vi "Create Unique File.vi"(8 "error in (no error)":errorcluster, 11 "appended path":path) -> (0 "error out":errorcluster, 3 "Byte Stream File out":refnum<file>)   [LabVIEW 2020, in "Global_logger.lvlib"]
uses:
  Global_logger.lvlib
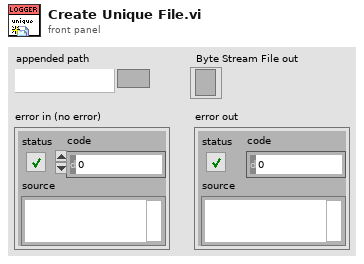
[diagram p1: front panel]
types:
  T1 = enum16{"open", "replace", "create", "open or create", "replace or create", "replace or create with confirmation"}
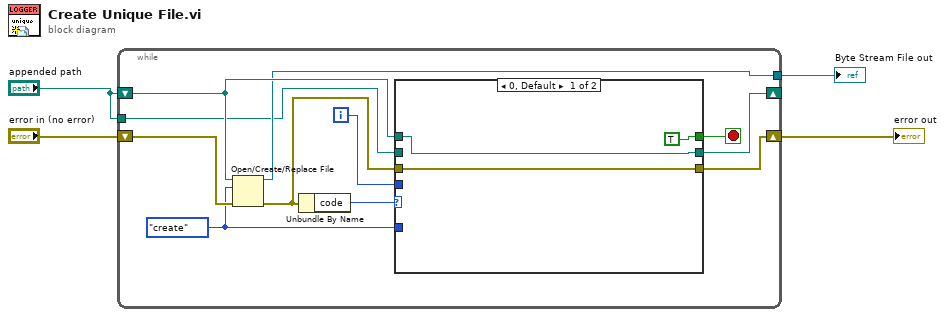
[diagram p0: block diagram]
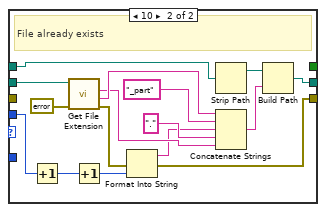
[diagram p2: hidden frame]
diagram:
  n1 = while {
    tunnel: [w7] -> w4
    shift-right: [w13] -> w3
    shift-left: "error in (no error)" -> [w15]
    shift-right: [w8] -> _
    shift-left: "appended path" -> [w11]
    tunnel: "appended path" -> [w5]
    i -> [w6]
    stop <- w9 stop-if-true
    w10 = T1."create" ("operation (0:open)")
    n2 = Open/Create/Replace File(file path (use dialog)=w11, error in=w15, operation (0:open)=w10) -> (refnum out=w7:refnum<file>, error out=w12:errorcluster)  [unwired: 3 in, 1 out]
    n3 = Unbundle By Name(w12) -> ("code"=w14:i32)
    n4 = case shown="0, Default" w14 {
      tunnel: [w18 w22] -> w13
      tunnel: w12 -> [w18 _]
      tunnel: w11 -> [w16 w27]
      tunnel: w10 -> [_ _]
      tunnel: [TRUE _] -> w9
      tunnel: [w16 w28] -> w8
      tunnel: w6 -> [_ w25]
      tunnel: w5 -> [_ w20]
      frame 0, Default {
      }
      frame 10 {
        # "File already exists"
        n5 = Increment(x=w25) -> (x+1=w21:i32)
        n6 = call <vilib>:"Get File Extension.vi"("error in (no error)"=errorcluster {"status"=FALSE, "code"=0, "source"=""} ("error in"), "file"=w20) -> ("error out"=w23:errorcluster, "filename without extension"=w33:string, "lowercase file extension"=w30:string)  [unwired: 5 in, 2 out]
        n7 = Increment(x=w21) -> (x+1=w19:i32)
        n8 = Format Into String(error in=w23, w19) -> (resulting string=w24:string, error out=w22:errorcluster)  [unwired: 2 in]
        n9 = Strip Path(path=w27) -> (stripped path=w26:path)  [unwired: 1 out]
        n10 = Concatenate Strings(w33, "_part" ("string"), w24, "." ("string"), w30) -> (w32:string)
        n11 = Build Path(base path=w26, name or relative path=w32) -> (appended path=w28:path)
      }
    }
  }
  "Byte Stream File out" <- w4
  "error out" <- w3
